vi "gun_tracking_mode_store.vi"(10 "data_store_mode":enum16{"Set", "Get"}(ring), 11 "gun tracking mode":T1) -> (3 "gun tracking mode":T1)   [LabVIEW 2011]
uses:
  gun_tracking_mode.ctl
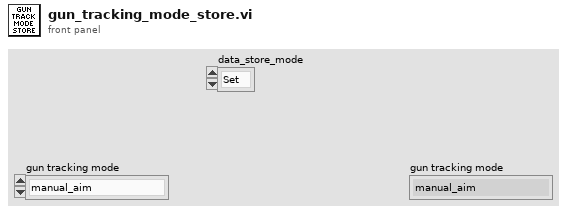
[diagram p1: front panel]
types:
  T1 = typedef "gun_tracking_mode.ctl" = enum16{"manual_aim", "auto_aim_camera", "preset_center_field", "preset_right_pocket", "preset_left_pocket", "align_center", "align_center_backwards", "auto_aim_key", "align_fold", "auton_custom", "preset_pass", "auto_aim_auton"}
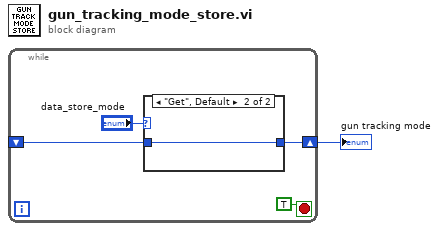
[diagram p0: block diagram]
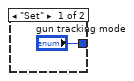
[diagram p2: hidden frame]
diagram:
  n1 = while {
    shift-right: [w3] -> w1
    shift-left: _ -> [w2]
    stop <- TRUE stop-if-true
    n2 = case shown="\"Get\", Default" "data_store_mode" {
      tunnel: ["gun tracking mode" w7] -> w3
      tunnel: w2 -> [_ w7]
      frame "Set" {
      }
      frame "Get", Default {
      }
    }
  }
  "gun tracking mode" <- w1
